vi "FTW-Endpoint-Destroy.vi"(0 "FTW Endpoint":refnum<class "FTW-Endpoint-TCP.lvclass">, 5 "Force Destroy":bool, 11 "error in":errorcluster) -> (15 "error out":errorcluster)   [LabVIEW 2015, in "FTW-Endpoint-TCP.lvclass"]
uses:
  FTW-Endpoint-TCP.lvclass
  FTW-Endpoint-TCP.lvclass/FTW-Endpoint-TCP.ctl
  Endpoint/FTW-Endpoint.lvclass
panel:
  # "Inputs"
  # "Outputs"
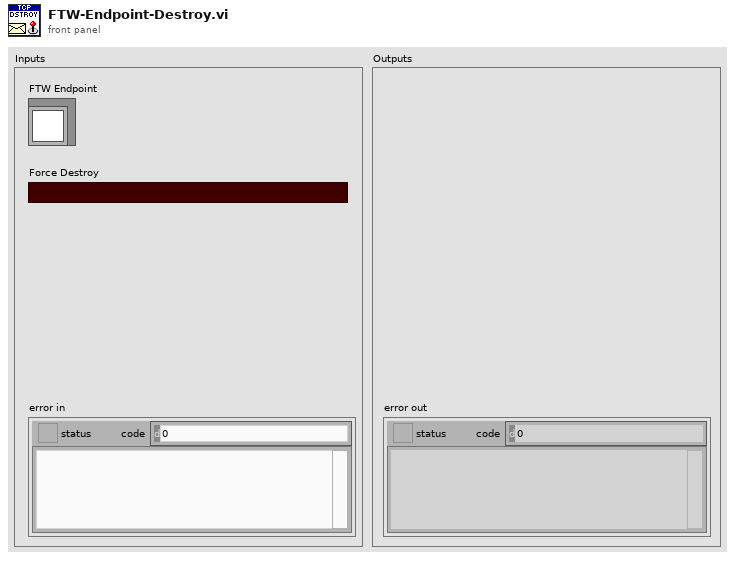
[diagram p1: front panel]
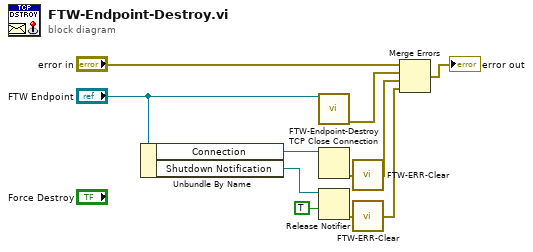
[diagram p0: block diagram]
diagram:
  n1 = Unbundle By Name("FTW Endpoint") -> ("Connection"=w11:refnum<k5>, "Shutdown Notification"=w6:refnum<notifier>)
  n2 = call-parent "FTW-Endpoint-Destroy.vi"("FTW Endpoint"="FTW Endpoint") -> ("error out"=w1:errorcluster)  [unwired: 14 in]
  n3 = TCP Close Connection(connection ID=w11) -> (error out=w8:errorcluster)  [unwired: 2 in, 1 out]
  n4 = Release Notifier(notifier=w6, force destroy? (F)=TRUE) -> (error out=w5:errorcluster)  [unwired: 1 in, 2 out]
  n5 = call "FTW-ERR-Clear.vi"("error to snuff"=w8) -> ("no error"=w7:errorcluster)
  n6 = call "FTW-ERR-Clear.vi"("error to snuff"=w5) -> ("no error"=w4:errorcluster)
  n7 = Merge Errors("error in", w1, w7, w4) -> (→"error out":errorcluster)
